vi "Handle Nested Status.vi"(8 "error in (no error)":errorcluster, 9 "Actor Error":errorcluster, 10 "State":T1, 11 "Actor Status Handler in":refnum<class "Actor Status Handler.lvclass">) -> (0 "error out":errorcluster, 3 "Actor Status Handler out":refnum<class "Actor Status Handler.lvclass">)   [LabVIEW 2022 SP3, in "Artifex.lvlib" / "Actor Status Handler.lvclass"]
uses:
  Actor Status Handler.lvclass
  Actor State.ctl
  Artifex.lvlib
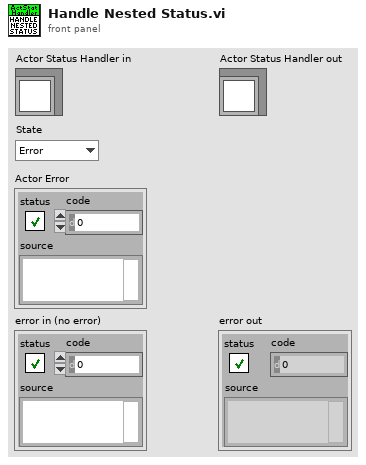
[diagram p1: front panel]
types:
  T1 = typedef "Artifex.lvlib/Actor State.ctl" = enum16{"Error", "Initialized", "Started", "Closing", "Closed"}
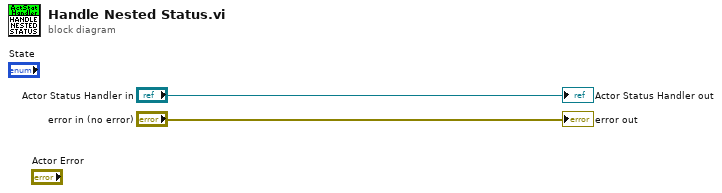
[diagram p0: block diagram]
diagram:
  "error out" <- "error in (no error)"
  "Actor Status Handler out" <- "Actor Status Handler in"
